vi "Generate write queue item.vi"(8 "error in (no error)":errorcluster, 10 "Request ID":u64, 11 "Subscribe JSON in":refnum<class "Subscribe JSON.lvclass">) -> (0 "error out":errorcluster, 2 "Write queue item":T1, 3 "Subscribe JSON out":refnum<class "Subscribe JSON.lvclass">)   [LabVIEW 2020, in "wamplv.lvlib" / "Subscribe JSON.lvclass"]
uses:
  Subscribe JSON.lvclass
  WAMP Client/Private/TypeDef/Write queue item.ctl
  TypeDefs/Transport type.ctl
  Subscribe JSON.lvclass/Subscribe JSON.ctl
  TypeDefs/WAMP Message Codes.ctl
  d3498a32-754b-4c76-a8e3-3724ae73477f.vi
  wamplv.lvlib
  Utils/Utils.lvclass
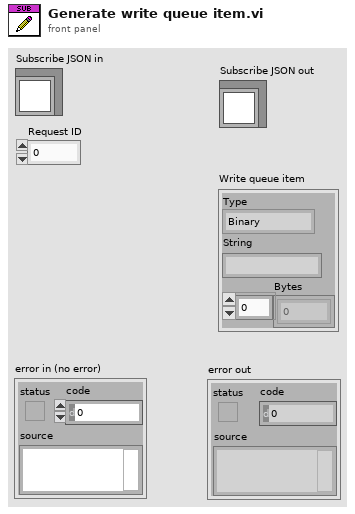
[diagram p1: front panel]
types:
  T1 = typedef "wamplv.lvlib/Write queue item.ctl" = cluster{"Type":T2, "String":string, "Bytes":u8[]}
  T2 = typedef "wamplv.lvlib/Transport type.ctl" = enum16{"Binary", "Text"}
  T3 = typedef "wamplv.lvlib/WAMP Message Codes.ctl" = enum8{"HELLO", "WELCOME", "CHALLENGE", "AUTHENTICATE", "ABORT", "GOODBYE", "ERROR", "PUBLISH", "PUBLISHED", "SUBSCRIBE", "SUBSCRIBED", "UNSUBSCRIBE", "UNSUBSCRIBED", "EVENT", "CALL", "RESULT", "REGISTER", "REGISTERED", "UNREGISTER", "UNREGISTERED", "INVOCATION", "YIELD"}
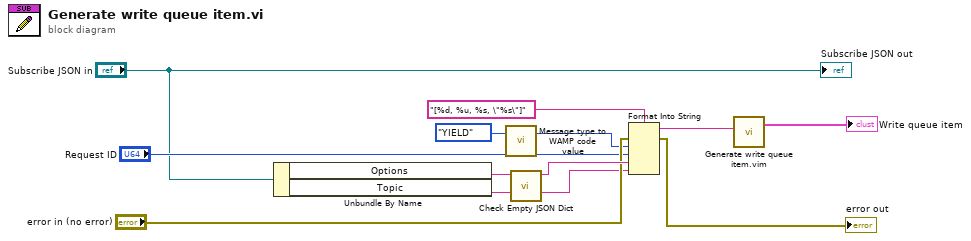
[diagram p0: block diagram]
diagram:
  n1 = Unbundle By Name("Subscribe JSON in") -> ("Options"=w4:string, "Topic"=w3:string)
  n2 = call "Message type to WAMP code value.vi"("Message Type"=WAMP_Message_Codes."YIELD" ("Message Codes")) -> ("WAMP Numeric value"=w7:u8)  [unwired: 2 in]
  n3 = call "Check Empty JSON Dict.vi"("JSON in"=w4) -> ("JSON out"=w11:string)  [unwired: 10 in]
  n4 = Format Into String(format string="[%d, %u, %s, \"%s\"]" ("element"), error in="error in (no error)", w7, "Request ID", w11, w3) -> (resulting string=w2:string, error out=→"error out":errorcluster)  [unwired: 1 in]
  n5 = call "Generate write queue item.vim"("Input"=w2) -> ("Ouput"=→"Write queue item":T1)  [unwired: 2 in]
  "Subscribe JSON out" <- "Subscribe JSON in"
